vi "LoadLegacyPalpation.vi"(8 "error in (no error)":errorcluster, 11 "File path":path) -> (0 "error out":errorcluster, 3 "Palpation":cluster{"Right":string, "Left":string})   [LabVIEW 2013, in "main.lvlib"]
uses:
  main.lvlib
  Globals/DataPathGlobalVariable.vi
  <userlib>/_OpenG.lib/file/file.llb/File Exists - Scalar__ogtk.vi
  <vilib>/Utility/file.llb/Read From Spreadsheet File (string).vi
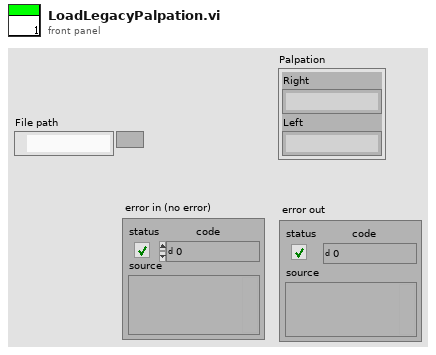
[diagram p1: front panel]
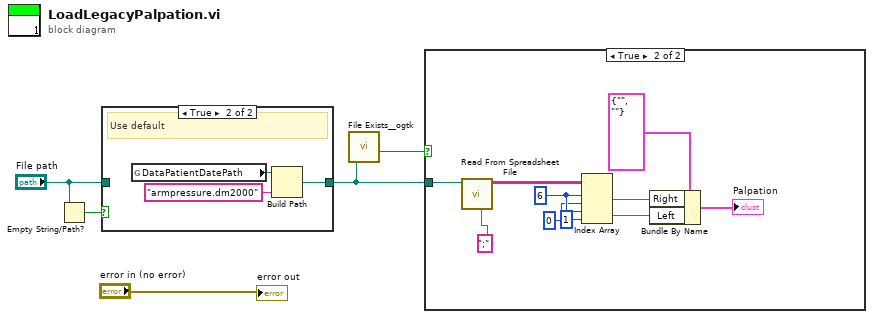
[diagram p0: block diagram]
diagram:
  n1 = Empty String/Path?(string/path="File path") -> (empty?=w3:bool)
  n2 = case shown="True" w3 {
    tunnel: [w6 w7] -> w4
    tunnel: "File path" -> [w6 _]
    frame False {
    }
    frame True {
      # "Use default"
      n3 = global read "DataPathGlobalVariable.vi" "DataPatientDatePath"() -> (w9:path)
      n4 = Build Path(base path=w9, name or relative path="armpressure.dm2000") -> (appended path=w7:path)
    }
  }
  n5 = call-poly <userlib>:"File Exists__ogtk.vi"("file path"=w4) -> ("exists"=w5:bool)  [unwired: 6 in, 1 out]
  n6 = case shown="True" w5 {
    tunnel: w4 -> [_ w18]
    frame False {
    }
    frame True {
      w17 = 6 ("index (row)")
      n7 = call-poly <vilib>:"Read From Spreadsheet File.vi"("delimiter (\\t)"=";" ("delimiter (\\t)"), "file path (dialog if empty)"=w18) -> ("all rows"=w14:string[][])  [unwired: 5 in, 4 out]
      n8 = Index Array(array=w14, index (row) #1=w17, index (col) #1=0 ("disabled index (col)"), index (row) #2=w17, index (col) #2=1 ("disabled index (col)")) -> (element #1=w13:string, element #2=w12:string)
      n9 = Bundle By Name(cluster=cluster{"Right":string, "Left":string} {"Right"="", "Left"=""}, "Right"=w13, "Left"=w12) -> (→"Palpation":cluster{"Right":string, "Left":string})
    }
  }
  "error out" <- "error in (no error)"
